vi "OnlyKeepCircularDepedentItems.vi"(9 "IgnoreLibrariesInCircularDependencies(True)":bool=TRUE, 11 "LibraryDependency In":map{path, T1}(c390)) -> (3 "LibraryDependency Out":map{path, T1}(c390))   [LabVIEW 2020, in "DependencyChecker.lvlib"]
uses:
  DependencyChecker.lvlib
  LibraryDependentInfo.vi
  <vilib>/Utility/lvfile.llb/FT_FileTypes.ctl
  <vilib>/Utility/lvfile.llb/NI_FileType.lvlib
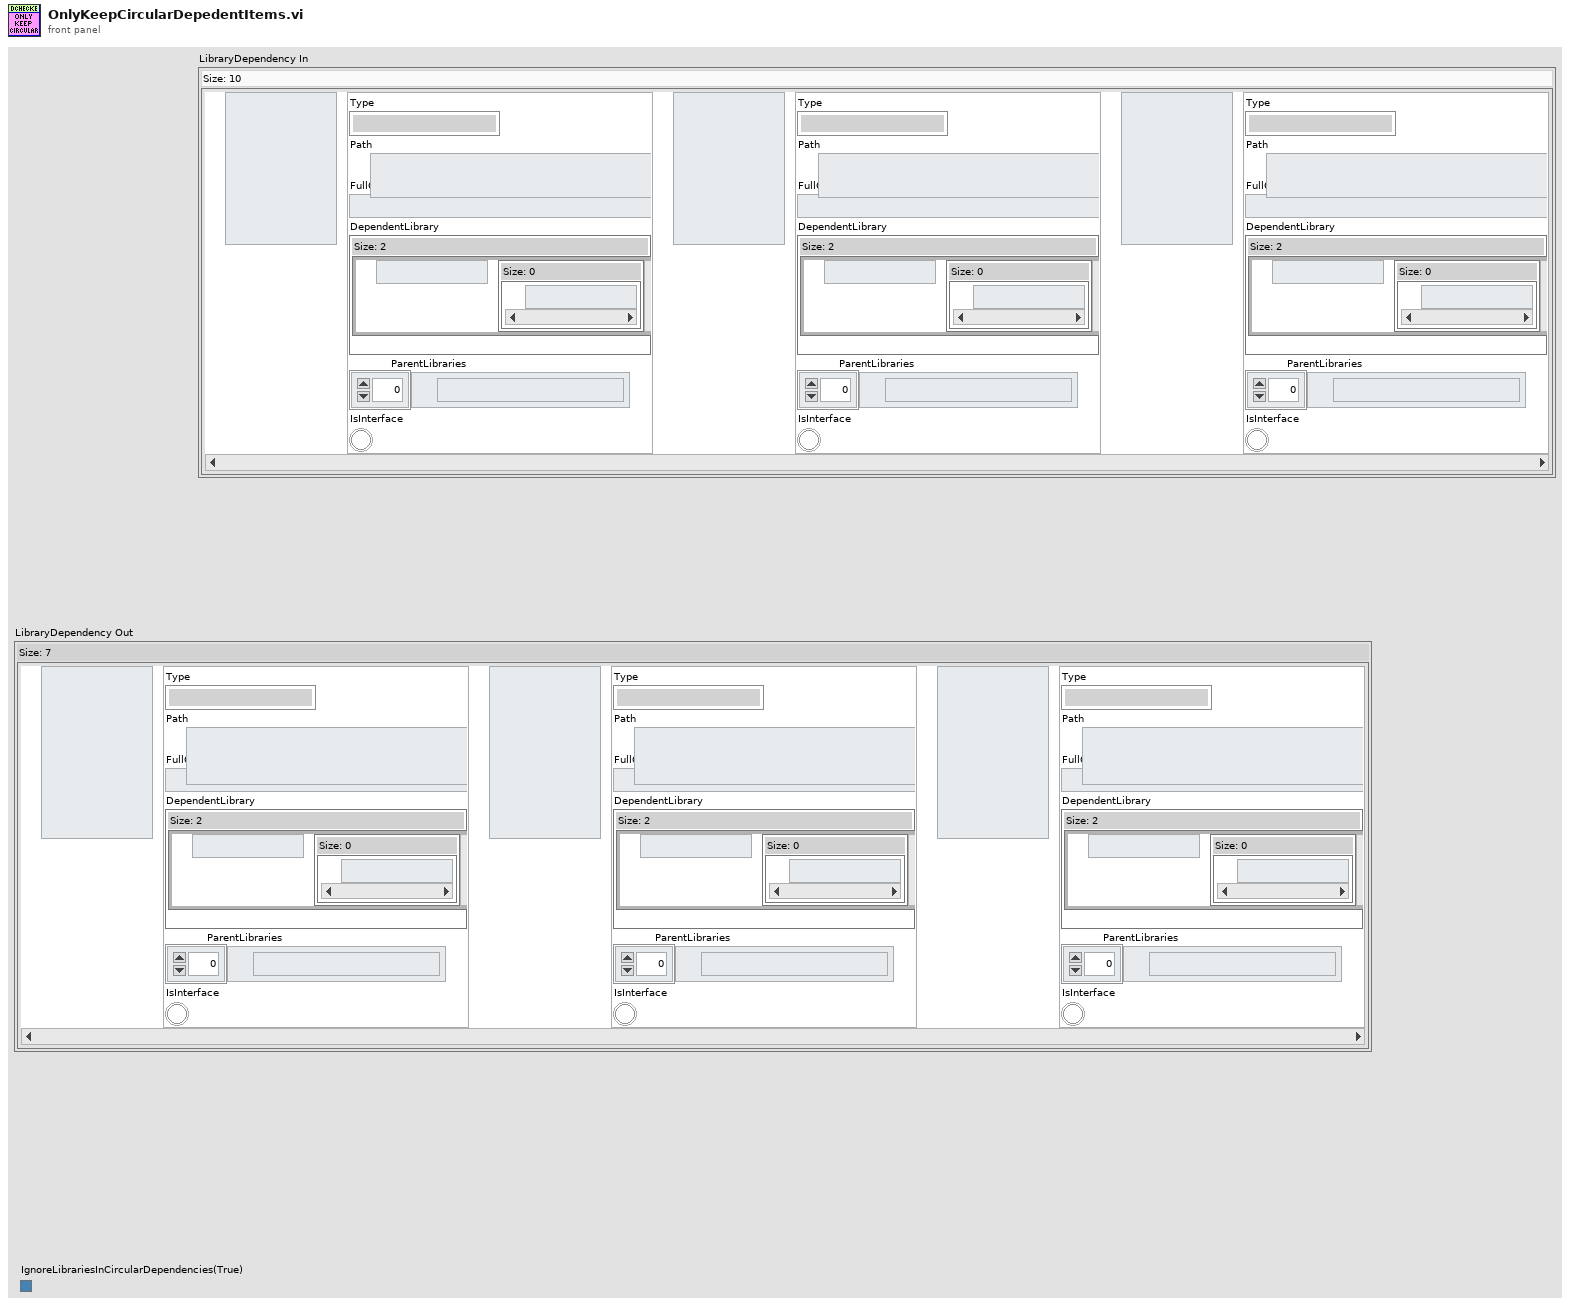
[diagram p1: front panel]
types:
  T1 = typedef "DependencyChecker.lvlib/LibraryDependentInfo.vi" = cluster{"Type":T2, "Path":path, "FullQualifierName":string, "DependentLibrary":map{path, set{path}}, "ParentLibraries":path[], "IsInterface":bool}
  T2 = typedef "NI_FileType.lvlib/FT_FileTypes.ctl" = enum32{"Invalid file/path", "Unknown type", "Instrument", "Control", "Polymorphic VI", "Project", "Library", "LVClass", "XControl", "XNode", "CIN", "Run-time menu", "Palette menu", "LLB", "Shortcut", "Directory", "Class Private Data Control", "Statechart", "MathScript .m file", "Ladder Diagram", "LVLibp"}
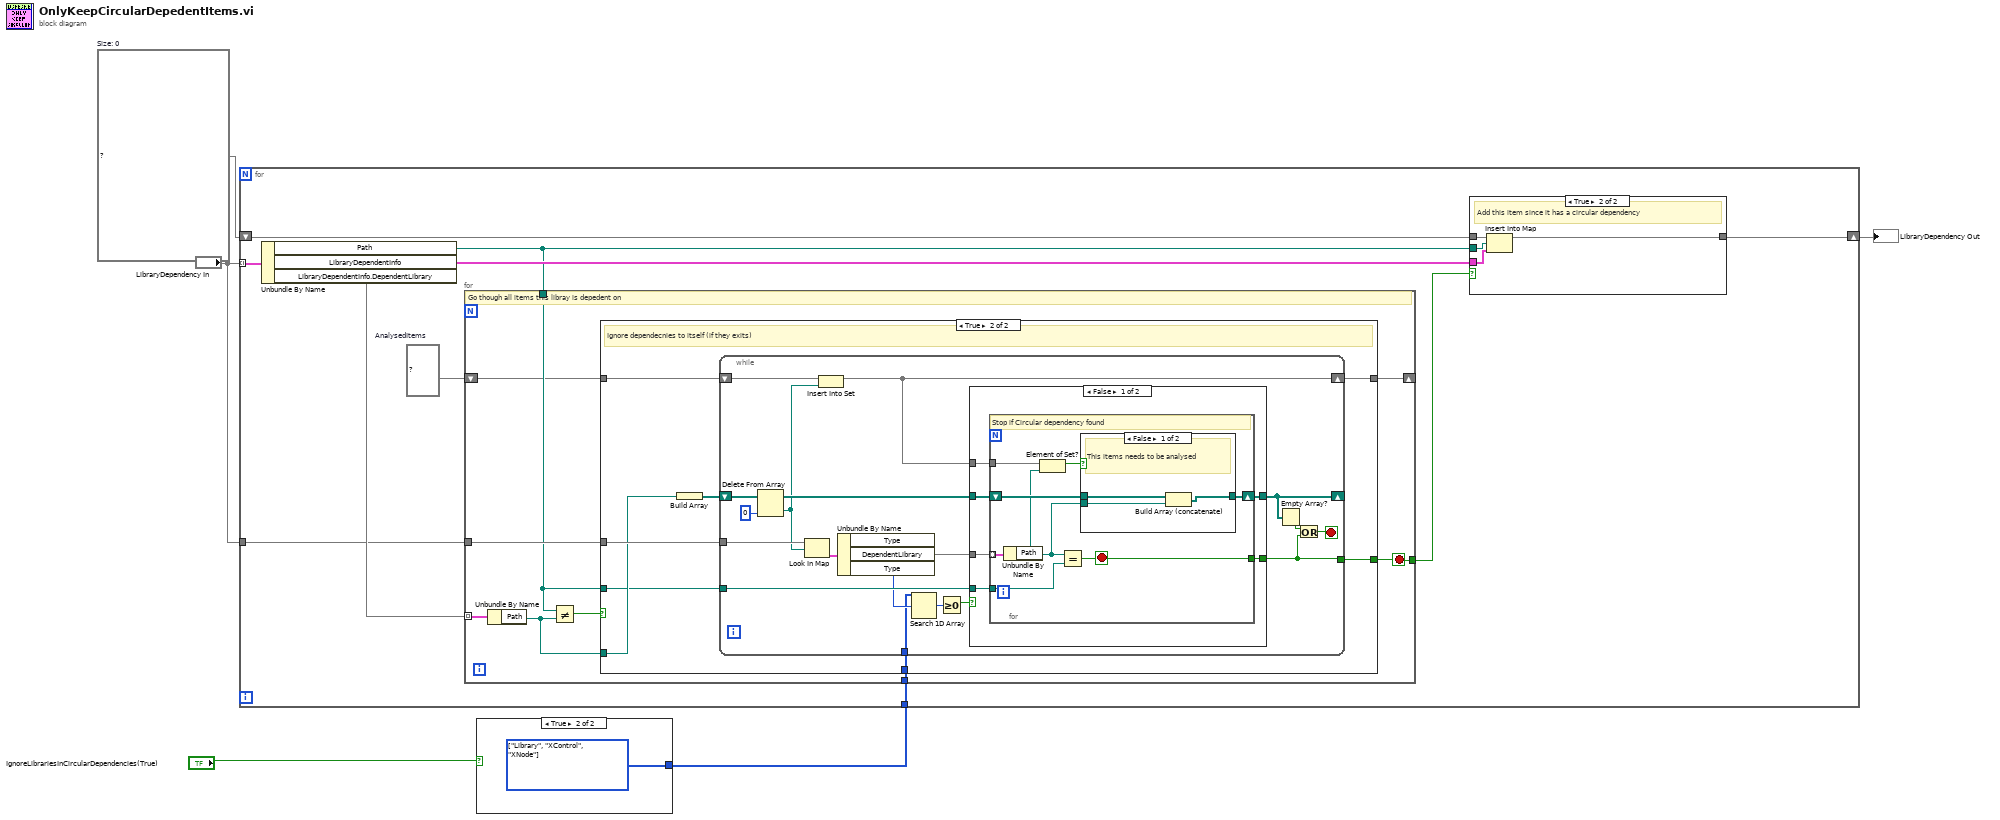
[diagram p0: block diagram]
diagram:
  w4 = map{path, T1} {}  # Size: 0
  n1 = case shown="True" "IgnoreLibrariesInCircularDependencies(True)" {
    tunnel: [_ w6] -> w1
    frame False {
    }
    frame True {
      w6 = T2[] [enum."Library", enum."XControl", enum."XNode"] items=["Invalid file/path", "Unknown type", "Instrument", "Control", "Polymorphic VI", "Project", "Library", "LVClass", "XControl", "XNode", "CIN", "Run-time menu", "Palette menu", "LLB", "Shortcut", "Directory", "Class Private Data Control", "Statechart", "MathScript .m file", "Ladder Diagram", "LVLibp"] ("y")
    }
  }
  n2 = for {
    tunnel: "LibraryDependency In" -> [w16] mode=indexing
    shift-right: [w15] -> w5
    shift-left: w4 -> [w11]
    tunnel: "LibraryDependency In" -> [w8]
    tunnel: w1 -> [w7]
    w9 = set{path} {}  # AnalysedItems
    n3 = Unbundle By Name(w16) -> ("Path"=w12:path, "LibraryDependentInfo"=w14:T1, "LibraryDependentInfo.DependentLibrary"=w13:map{path, set{path}})
    n4 = for {
      tunnel: w13 -> [w25] mode=indexing
      tunnel: w12 -> [w21]
      tunnel: w8 -> [w23]
      tunnel: [w20] -> w10
      shift-right: [w18] -> _
      shift-left: w9 -> [w19]
      tunnel: w7 -> [w17]
      stop <- w20 stop-if-true
      # "Go though all items this libray is depedent on"
      n5 = Unbundle By Name(w25) -> ("Path"=w22:path)
      n6 = Not Equal?(x=w21, y=w22) -> (x != y?=w24:bool)
      n7 = case shown="True" w24 {
        tunnel: w23 -> [_ w34]
        tunnel: w22 -> [_ w33]
        tunnel: w21 -> [_ w31]
        tunnel: [_ w30] -> w20
        tunnel: w19 -> [w26 w29]
        tunnel: [w26 w28] -> w18
        tunnel: w17 -> [_ w27]
        frame False {
          # "Ignore Self depedency (if exists)"
        }
        frame True {
          # "Ignore dependecnies to itself (if they exits)"
          n8 = Build Array(w33) -> (w32:path[])
          n9 = while {
            tunnel: w34 -> [w52]
            shift-right: [w42] -> _
            shift-left: w32 -> [w49]
            tunnel: w31 -> [w47]
            tunnel: [w40] -> w30
            shift-right: [w43] -> w28
            shift-left: w29 -> [w45]
            tunnel: w27 -> [w37]
            stop <- w39 stop-if-true
            n10 = Delete From Array(array=w49, index=0) -> (deleted portion=w44:path, array with subset deleted=w46:path[])  [unwired: 1 in]
            n11 = Look In Map(map=w52, key=w44) -> (value=w51:T1)  [unwired: 1 in, 1 out]
            n12 = Insert Into Set(10:w44, 11:w45) -> (3:w43:set{path})  [unwired: 1 out]
            n13 = Unbundle By Name(w51) -> ("DependentLibrary"=w50:map{path, set{path}}, "Type"=w38:T2)  [unwired: 1 out]
            n14 = Search 1D Array(1D array=w37, element=w38) -> (index of element=w36:i32)  [unwired: 1 in]
            n15 = Greater Or Equal To 0?(x=w36) -> (x >= 0?=w35:bool)
            n16 = case shown="False" w35 {
              tunnel: w50 -> [w58 _]
              tunnel: w47 -> [w57 _]
              tunnel: w46 -> [w56 w71]
              tunnel: w43 -> [w55 _]
              tunnel: [w54 w71] -> w42
              tunnel: [w53 _] -> w40
              frame False {
                n17 = for {
                  tunnel: w58 -> [w66] mode=indexing
                  tunnel: w57 -> [w65]
                  tunnel: [w64] -> w53
                  shift-right: [w60] -> w54
                  shift-left: w56 -> [w61]
                  tunnel: w55 -> [w63]
                  stop <- w64 stop-if-true
                  # "Stop if Circular dependency found"
                  n18 = Unbundle By Name(w66) -> ("Path"=w59:path)
                  n19 = Element of Set?(10:w59, 11:w63) -> (3:w62:bool)
                  n20 = Equal?(x=w59, y=w65) -> (x = y?=w64:bool)
                  n21 = case shown="False" w62 {
                    tunnel: w61 -> [w69 w70]
                    tunnel: [w68 w70] -> w60
                    tunnel: w59 -> [w67 _]
                    frame False {
                      # "This items needs to be analysed"
                      n22 = Build Array (concatenate)(w69, w67) -> (w68:path[])
                    }
                    frame True {
                      # "This item has already been analysed"
                    }
                  }
                }
              }
              frame True {
                # "Ingore this type"
              }
            }
            n23 = Empty Array?(array=w42) -> (empty?=w41:bool)
            n24 = Or(x=w41, y=w40) -> (x .or. y?=w39:bool)
          }
        }
      }
    }
    n25 = case shown="True" w10 {
      tunnel: w11 -> [w72 w76]
      tunnel: w12 -> [_ w74]
      tunnel: [w72 w75] -> w15
      tunnel: w14 -> [_ w73]
      frame False {
        # "Not in a circular dependency"
      }
      frame True {
        # "Add this item since it has a circular dependency"
        n26 = Insert Into Map(map in=w76, key=w74, value=w73) -> (map out=w75:map{path, T1})  [unwired: 2 out]
      }
    }
  }
  "LibraryDependency Out" <- w5
